vi "ResortCoeffs.vi"(8 "error in (no error)":errorcluster, 11 "CoeFile in":refnum<class "CoeFile.lvclass">) -> (0 "error out":errorcluster, 3 "CoeFile out":refnum<class "CoeFile.lvclass">)   [LabVIEW 2025, in "CoeFile.lvclass"]
uses:
  CoeFile.lvclass
  CoeFile.lvclass/CoeFile.ctl
  <userlib>/_OpenG.lib/error/error.llb/openg_error.lvlib
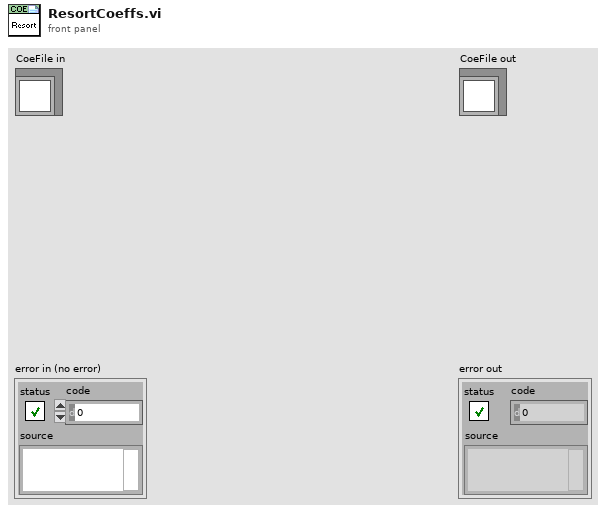
[diagram p1: front panel]
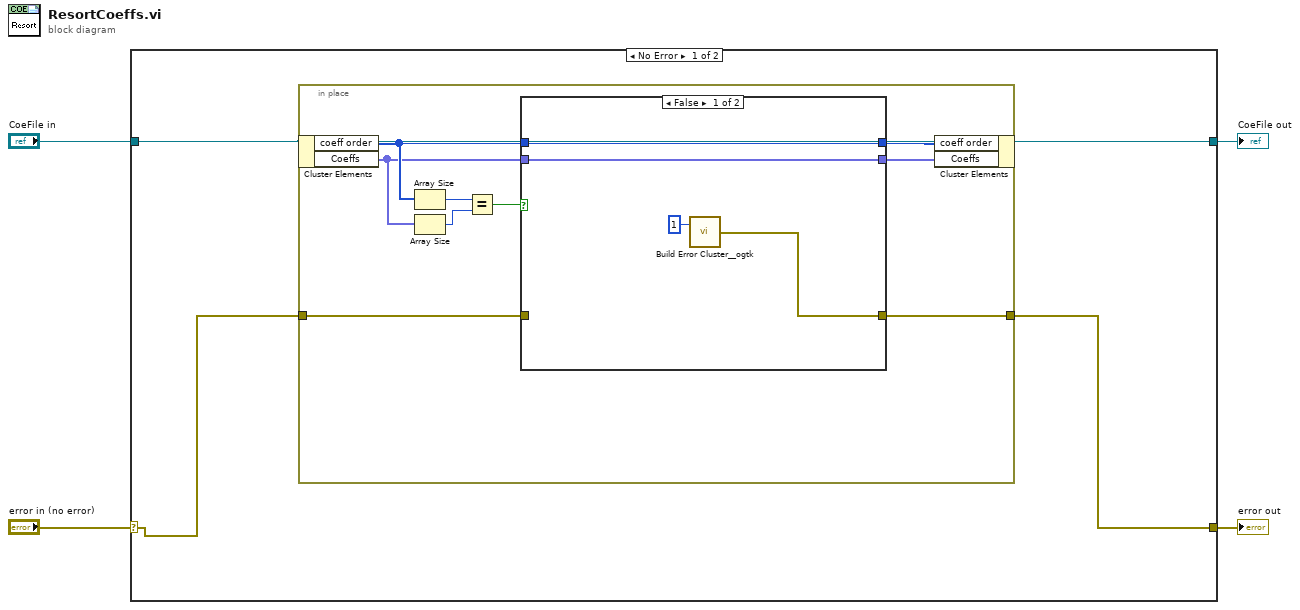
[diagram p0: block diagram]
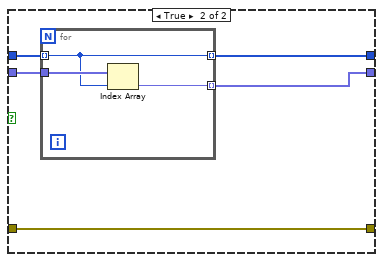
[diagram p2: hidden frame]
diagram:
  n1 = case shown="No Error" "error in (no error)" {
    selector: "error in (no error)" -> [w5 w30]
    tunnel: [w6 w30] -> w3
    tunnel: [w7 w29] -> w1
    tunnel: "CoeFile in" -> [w7 w29]
    frame No Error {
      n2 = in-place {
        in-place-border: [w9] -> w6
        in-place-border: w5 -> [w8]
        n3 = in-place-cluster #1(w7) -> ("coeff order"=w14:i32[], "Coeffs"=w13:fxp<+/-,18,18>[])
        n4 = Array Size(array=w14) -> (size(s)=w12:i32)
        n5 = Array Size(array=w13) -> (size(s)=w11:i32)
        n6 = Equal?(x=w12, y=w11) -> (x = y?=w10:bool)
        n7 = case shown="False" w10 {
          tunnel: [w19 w25] -> w16
          tunnel: [w20 w24] -> w15
          tunnel: w14 -> [w20 w23]
          tunnel: w13 -> [w19 w22]
          tunnel: [w17 w21] -> w9
          tunnel: w8 -> [_ w21]
          frame False {
            n8 = call <userlib>:"Build Error Cluster__ogtk.vi"("code"=1) -> ("error out"=w17:errorcluster)  [unwired: 1 in]
          }
          frame True {
            n9 = for {
              tunnel: w23 -> [w26] mode=indexing
              tunnel: w22 -> [w28]
              tunnel: [w27] -> w25 mode=indexing
              tunnel: [w26] -> w24 mode=indexing
              n10 = Index Array(array=w28, index=w26) -> (element=w27:fxp<+/-,18,18>)
            }
          }
        }
        n11 = in-place-cluster #1("coeff order"=w15, "Coeffs"=w16) -> ()  [unwired: 1 out]
      }
    }
    frame Error {
    }
  }
  "error out" <- w3
  "CoeFile out" <- w1
